vi "Apply Selected Labels to Control.vi"(8 "error in (no error)":errorcluster, 10 "Alternate Text Select (0)":i32, 11 "Array in":refnum<class "Array.lvclass">) -> (0 "error out":errorcluster, 3 "Array out":refnum<class "Array.lvclass">)   [LabVIEW 2017, in "Localization.lvlib" / "Array.lvclass"]
doc: "Use the information in the class to apply the selected alternate text from the Additional Labels to the control.\n\nChoose Movement Consulting, LLC"
uses:
  Array.lvclass
  C:/Apps/CMC/OpenSource/Localization/Control Info/Control Info.lvclass
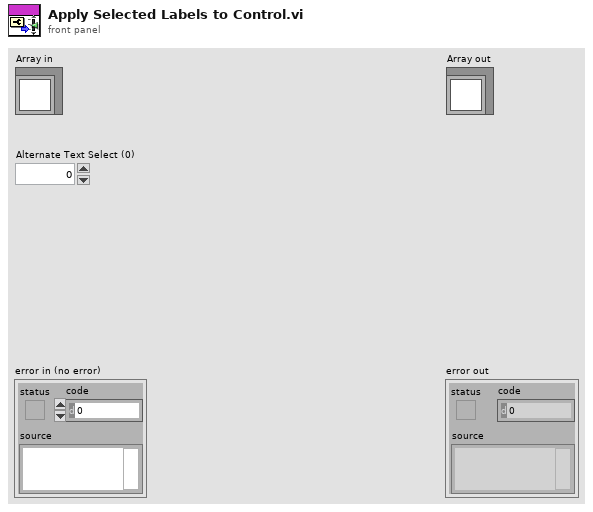
[diagram p1: front panel]
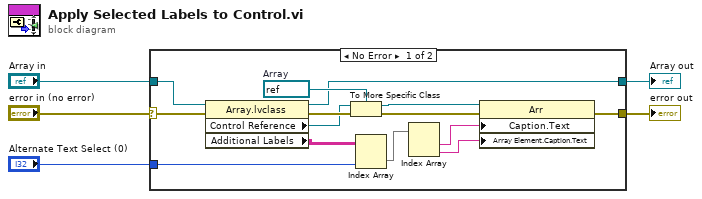
[diagram p0: block diagram]
diagram:
  n1 = case shown="No Error" "error in (no error)" {
    selector: "error in (no error)" -> [w14 w21]
    tunnel: "Array in" -> [w13 w20]
    tunnel: [w8 w21] -> w4
    tunnel: [w7 w20] -> w3
    tunnel: "Alternate Text Select (0)" -> [w11 _]
    frame No Error {
      w19 = refnum<vi> refnum  # Array
      n2 = property class="Array.lvclass"(reference=w13, error in=w14) -> (reference out=w7:refnum<class "Array.lvclass">, error out=w16:errorcluster, "Control Reference"=w15:refnum<vi>, "Additional Labels"=w12:string[][])
      n3 = To More Specific Class(target class=w19, reference=w15, error in=w16) -> (specific class reference=w18:refnum<vi>, error out=w17:errorcluster)
      n4 = Index Array(array=w12, index (col)=w11) -> (element=w9:string[])  [unwired: 1 in]
      n5 = Index Array(array=w9) -> (element #1=w10:string, element #2=w6:string)  [unwired: 2 in]
      n6 = property class="Arr"(reference=w18, error in=w17, "Caption.Text"=w10, "Array Element.Caption.Text"=w6) -> (error out=w8:errorcluster)  [unwired: 1 out]
    }
    frame Error {
    }
  }
  "error out" <- w4
  "Array out" <- w3
